vi "GetType.vi"(8 "error in (no error)":errorcluster, 11 "Update_RawActPosition Msg":refnum<class "Update_RawActPosition Msg.lvclass">) -> (0 "error out":errorcluster, 2 "Data Sample":variant, 3 "Update_RawActPosition Msg":refnum<class "Update_RawActPosition Msg.lvclass">)   [LabVIEW 2015, in "CS++Motor.lvlib" / "Update_RawActPosition Msg.lvclass"]
uses:
  Update_RawActPosition Msg.lvclass
  Update_RawActPosition Msg.lvclass/Update_RawActPosition Msg.ctl
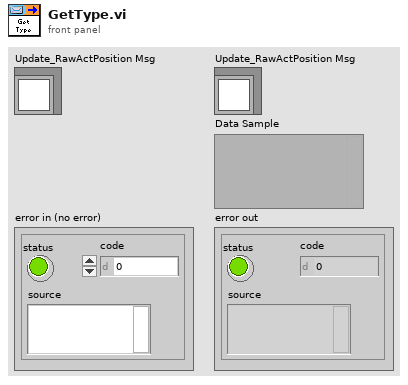
[diagram p1: front panel]
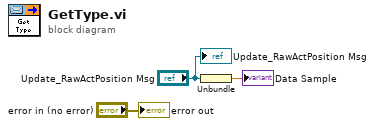
[diagram p0: block diagram]
diagram:
  n1 = Unbundle("Update_RawActPosition Msg") -> (→"Data Sample":dbl)
  "error out" <- "error in (no error)"
  "Update_RawActPosition Msg" <- "Update_RawActPosition Msg"
